vi "Lakeshore 370 - send GPIB cmd.vi"(8 "error in (no error)":errorcluster, 10 "Cmd string":string="GetTemp", 11 "Enum":enum16{"Sample stage", "Mixing chamber"}(ring)=enum."Mixing chamber") -> (0 "error out":errorcluster, 2 "Response":string)   [LabVIEW 2019]
doc: "Nicolas Weiss - EPFL - IPHYS 2019\n----\nThis VI sends the GPIB commands to the device (without performing syntax and in-range argument check).\nThus, the commands *must* first be checked by the \"Check and send command to corresponding device.vi\""
uses:
  _Global variables 1.vi
  <instrlib>/Lake Shore Cryotronics 370/Lake Shore Cryotronics 370.lvlib
panel:
  out "Arguments":string[](array[string])
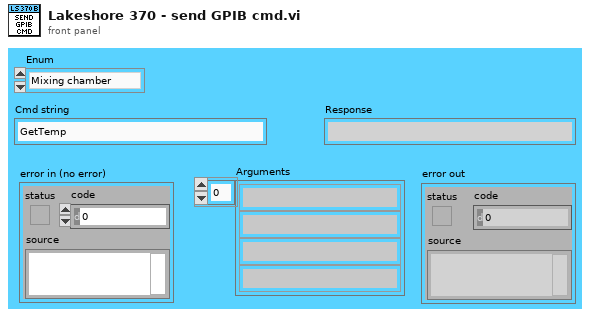
[diagram p1: front panel]
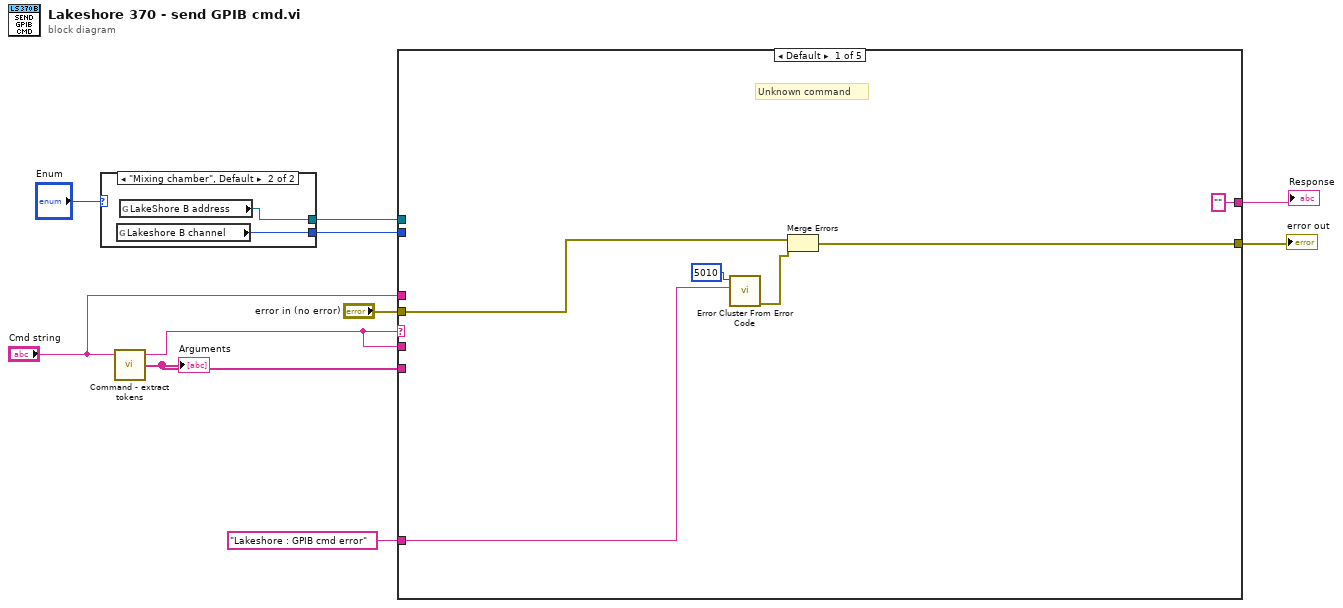
[diagram p0: block diagram]
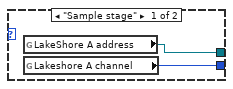
[diagram p2: hidden frame]
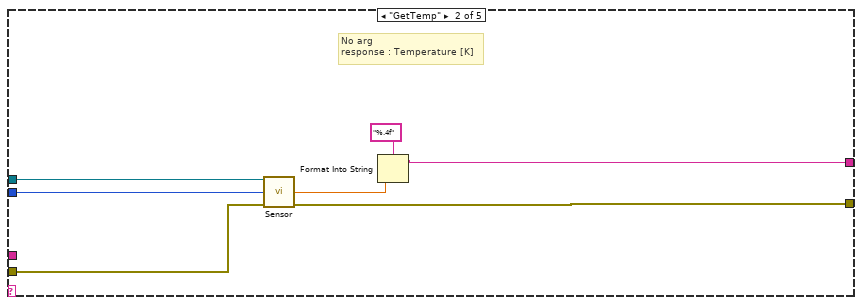
[diagram p3: hidden frame]
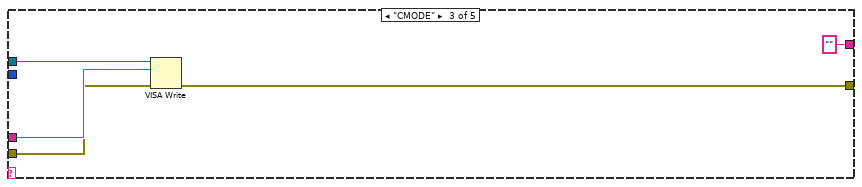
[diagram p4: hidden frame]
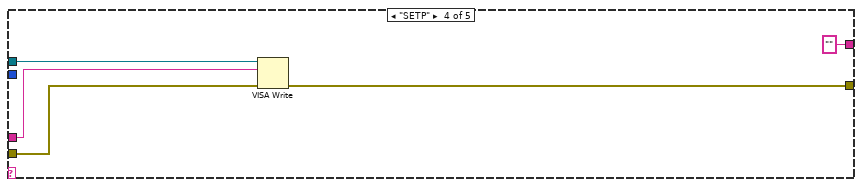
[diagram p5: hidden frame]
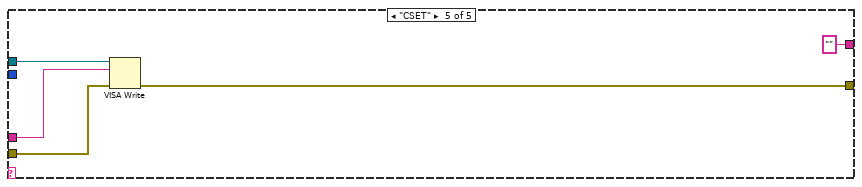
[diagram p6: hidden frame]
diagram:
  n1 = case shown="\"Mixing chamber\", Default" "Enum" {
    tunnel: [w11 w13] -> w1
    tunnel: [w12 w14] -> w5
    frame "Sample stage" {
      n2 = global read "_Global variables 1.vi" "LakeShore A address"() -> (w11:refnum<visa-resource-name>)
      n3 = global read "_Global variables 1.vi" "Lakeshore A channel"() -> (w12:u8)
    }
    frame "Mixing chamber", Default {
      n4 = global read "_Global variables 1.vi" "Lakeshore B channel"() -> (w14:u8)
      n5 = global read "_Global variables 1.vi" "LakeShore B address"() -> (w13:refnum<visa-resource-name>)
    }
  }
  n6 = call "Command - extract tokens.vi"("Cmd string"="Cmd string") -> ("Arguments"=w6:string[], "Command"=w3:string)  [unwired: 2 in, 1 out]
  "Arguments" <- w6
  n7 = case shown="Default" w3 {
    tunnel: w6 -> [_ _ _ _ _]
    tunnel: w1 -> [_ w27 w31 w35 w42]
    tunnel: "error in (no error)" -> [w15 w26 w30 w33 w40]
    tunnel: [w18 w25 w29 w36 w39] -> w9
    tunnel: ["" w22 "" "" ""] -> w8
    tunnel: "Lakeshore : GPIB cmd error" ("format string") -> [w17 _ _ _ _]
    tunnel: w5 -> [_ w21 _ _ _]
    tunnel: w3 -> [_ _ _ _ _]
    tunnel: "Cmd string" -> [_ _ w32 w34 w41]
    frame Default {
      # "Unknown command"
      n8 = call <vilib>:"Error Cluster From Error Code.vi"("error message (\"\")"=w17, "error code (0)"=5010) -> ("error out"=w20:errorcluster)  [unwired: 7 in]
      n9 = Merge Errors(w15, w20) -> (w18:errorcluster)
    }
    frame "GetTemp" {
      # "No arg\nresponse : Temperature [K]"
      n10 = call <instrlib>:"Sensor.vi"("VISA resource name"=w27, "Channel (1)"=w21, "error in (no error)"=w26) -> ("Kelvin Reading"=w24:dbl, "error out"=w25:errorcluster)  [unwired: 8 in, 3 out]
      n11 = Format Into String(format string="%.4f", w24) -> (resulting string=w22:string)  [unwired: 2 in, 1 out]
    }
    frame "CMODE" {
      n12 = VISA Write(VISA resource name=w31, write buffer=w32, error in (no error)=w30) -> (error out=w29:errorcluster)  [unwired: 2 out]
    }
    frame "SETP" {
      n13 = VISA Write(VISA resource name=w35, write buffer=w34, error in (no error)=w33) -> (error out=w36:errorcluster)  [unwired: 2 out]
    }
    frame "CSET" {
      n14 = VISA Write(VISA resource name=w42, write buffer=w41, error in (no error)=w40) -> (error out=w39:errorcluster)  [unwired: 2 out]
    }
  }
  "error out" <- w9
  "Response" <- w8
